vi "Filter Data.vi"(8 "error in":errorcluster, 9 "Record state change":bool=TRUE, 10 "Analyzed Data Sets":T1) -> (0 "error out":errorcluster, 1 "Send?":bool, 2 "Analyzed Data Sets Out":T1)   [LabVIEW 2018, in "File IO.lvlib"]
uses:
  File IO.lvlib
  Top Level/Shared Controls/Analyzed Data Sets.ctl
  Top Level/Shared Controls/All Data Cluster.ctl
  Top Level/Shared Controls/Acq Data.ctl
  Top Level/Shared Controls/Post-Analysis Data.ctl
  Top Level/Shared Controls/Calculated Data.ctl
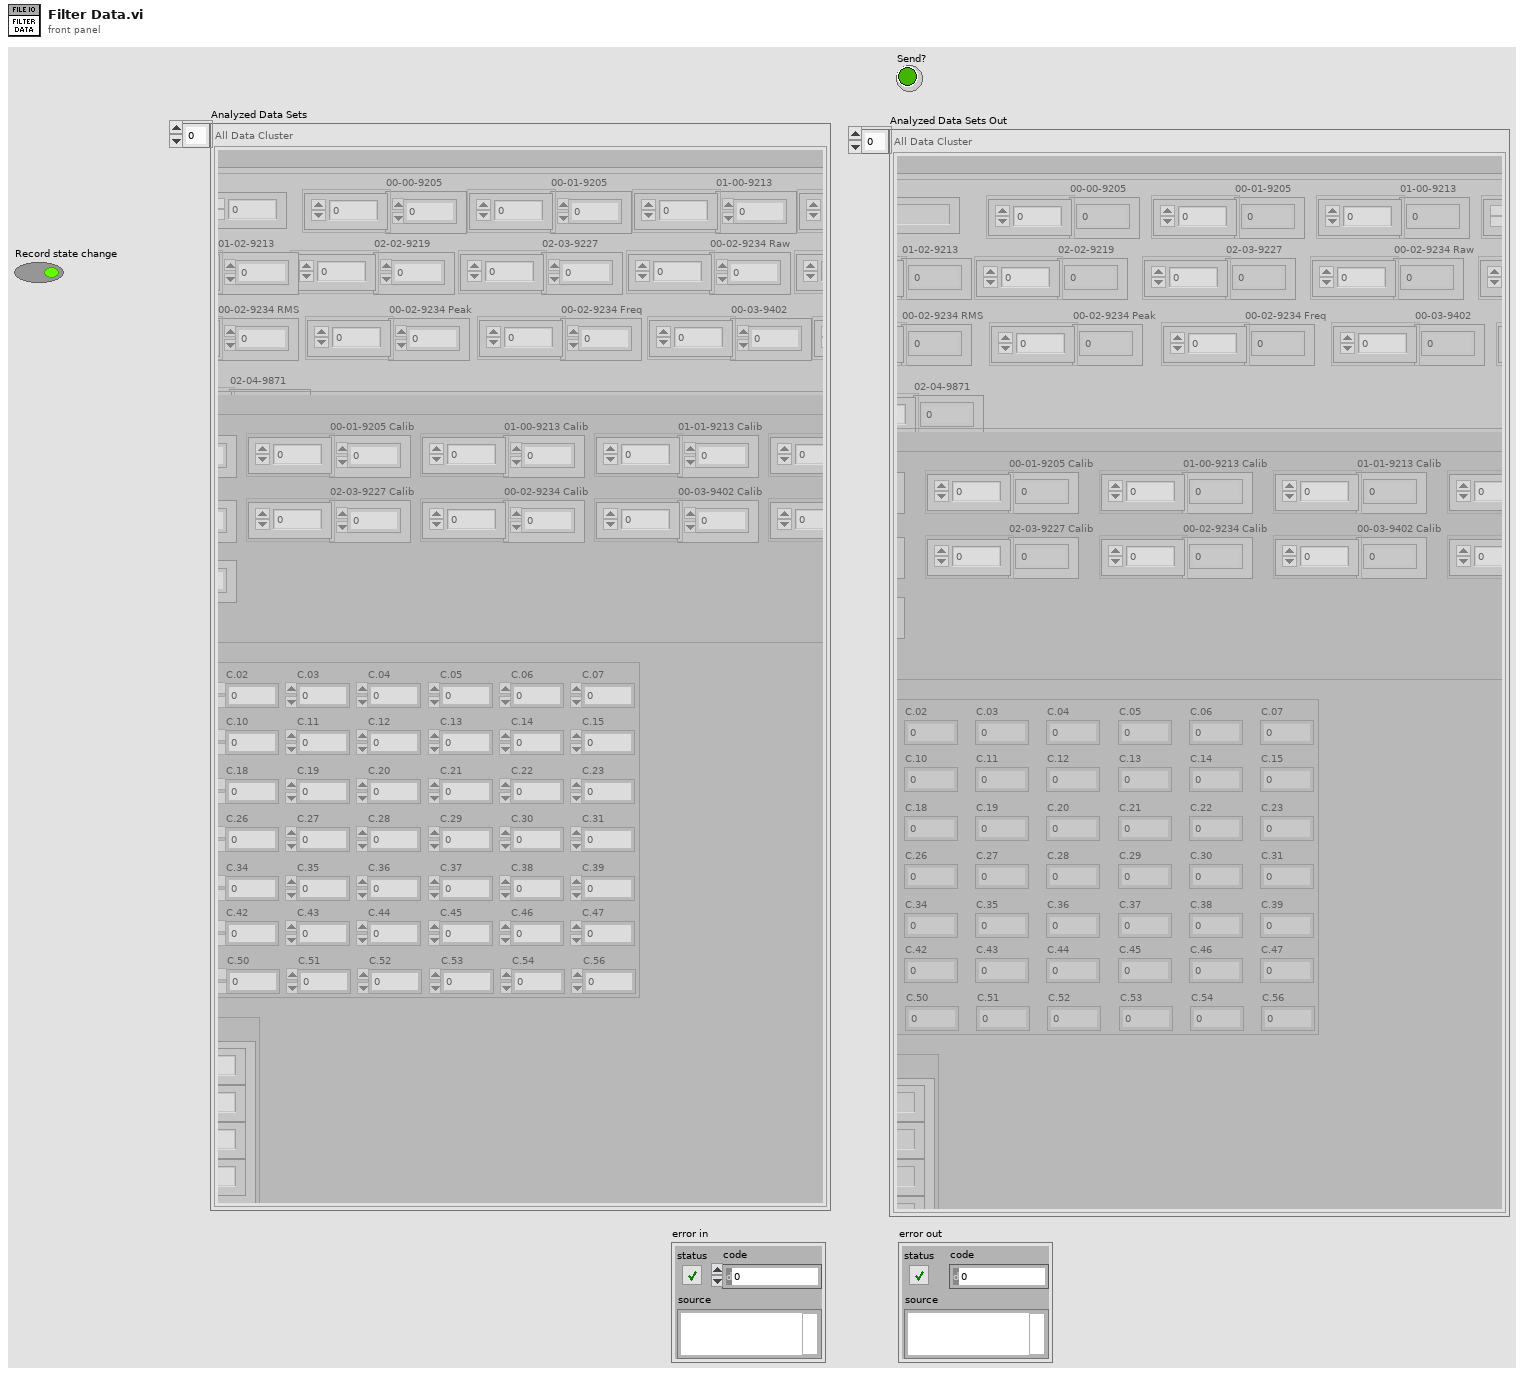
[diagram p1: front panel]
types:
  T1 = typedef "Analyzed Data Sets.ctl" = T2[]
  T2 = typedef "All Data Cluster.ctl" = cluster{"Acq Data":T3, "Post-Analysis Data":T4}
  T3 = typedef "Acq Data.ctl" = cluster{"Timestamp":timestamp, "Acq Period (ms)":i64, "00-00-9205":dbl[], "00-01-9205":dbl[], "01-00-9213":dbl[], "01-01-9213":dbl[], "01-02-9213":dbl[], "02-02-9219":dbl[], "02-03-9227":dbl[], "00-02-9234 Raw":dbl[], "00-02-9234 DC":dbl[], "00-02-9234 RMS":dbl[], "00-02-9234 Peak":dbl[], "00-02-9234 Freq":dbl[], "00-03-9402":dbl[], "02-05-9205":dbl[], "02-04-9871":dbl[]}
  T4 = typedef "Post-Analysis Data.ctl" = cluster{"Calibrated Data":cluster{"00-00-9205 Calib":dbl[], "00-01-9205 Calib":dbl[], "01-00-9213 Calib":dbl[], "01-01-9213 Calib":dbl[], "01-02-9213 Calib":dbl[], "02-02-9219 Calib":dbl[], "02-03-9227 Calib":dbl[], "00-02-9234 Calib":dbl[], "00-03-9402 Calib":dbl[], "02-05-9205 Calib":dbl[], "02-04-9871 2DArray":dbl[][]}, "Calculated Data":T5, "Indicator Data":cluster{"00-02-9234 Peak Vel (in/sec)":dbl[]}}
  T5 = typedef "Calculated Data.ctl" = cluster{"C.00":dbl, "C.01":dbl, "C.02":dbl, "C.03":dbl, "C.04":dbl, "C.05":dbl, "C.06":dbl, "C.07":dbl, "C.08":dbl, "C.09":dbl, "C.10":dbl, "C.11":dbl, "C.12":dbl, "C.13":dbl, "C.14":dbl, "C.15":dbl, "C.16":dbl, "C.17":dbl, "C.18":dbl, "C.19":dbl, "C.20":dbl, "C.21":dbl, "C.22":dbl, "C.23":dbl, "C.24":dbl, "C.25":dbl, "C.26":dbl, "C.27":dbl, "C.28":dbl, "C.29":dbl, "C.30":dbl, "C.31":dbl, "C.32":dbl, "C.33":dbl, "C.34":dbl, "C.35":dbl, "C.36":dbl, "C.37":dbl, "C.38":dbl, "C.39":dbl, "C.40":dbl, "C.41":dbl, "C.42":dbl, "C.43":dbl, "C.44":dbl, "C.45":dbl, "C.46":dbl, "C.47":dbl, "C.48":dbl, "C.49":dbl, "C.50":dbl, "C.51":dbl, "C.52":dbl, "C.53":dbl, "C.54":dbl, "C.56":dbl}
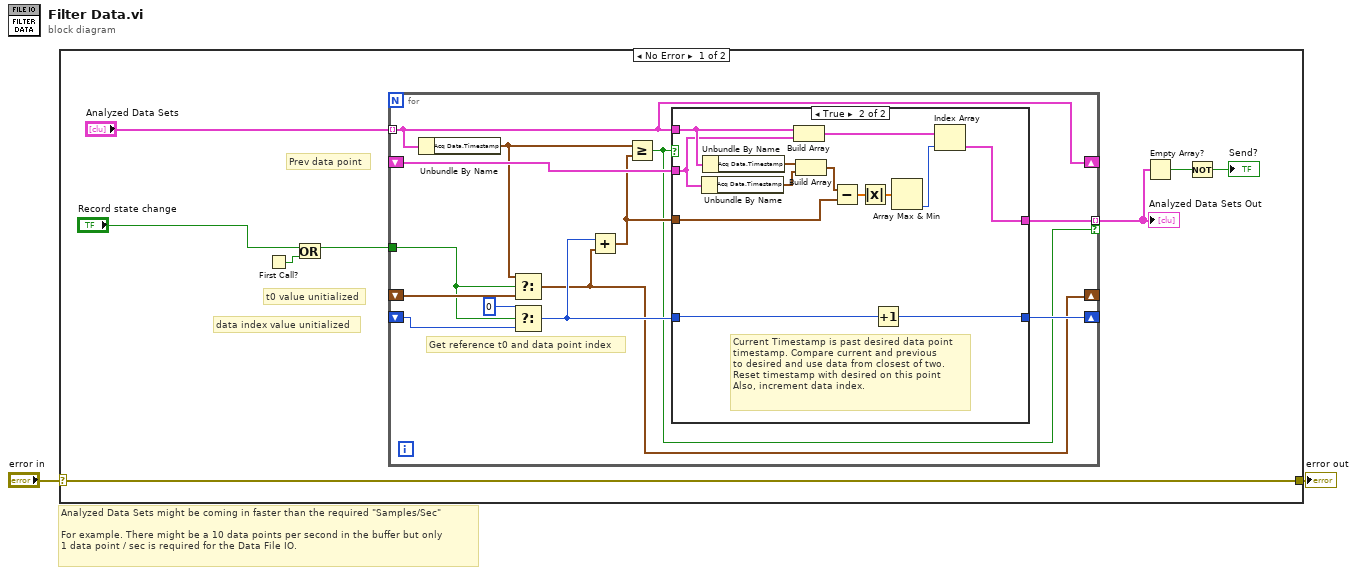
[diagram p0: block diagram]
diagram:
  # "Analyzed Data Sets might be coming in faster than the required \"Samples/Sec\"\n\nFor example. There might be a 10 data points per second in the buffer but only \n1 data point / sec is required for the Data File IO."
  n1 = case shown="No Error" "error in" {
    selector: "error in" -> [w3 w39]
    tunnel: [w3 w39] -> w1
    frame No Error {
      # "Prev data point"
      # "data index value unitialized"
      # "t0 value unitialized"
      n2 = First Call?() -> (First Call?: T/F=w5:bool)
      n3 = Or(x="Record state change", y=w5) -> (x .or. y?=w6:bool)
      n4 = for {
        tunnel: "Analyzed Data Sets" -> [w14] mode=indexing
        tunnel: w6 -> [w20]
        shift-right: [w12] -> _
        shift-left: _ -> [w23]
        shift-right: [w16] -> _
        shift-left: _ -> [w21]
        shift-right: [w14] -> _
        shift-left: _ -> [w19]
        tunnel: [w13] -> w4 mode=indexing if=w15
        # "Get reference t0 and data point index"
        n5 = Unbundle By Name(w14) -> ("Acq Data.Timestamp"=w11:timestamp)
        n6 = Select(t=w11, s=w20, f=w23) -> (s? t:f=w12:timestamp)
        n7 = Select(t=i64 0, s=w20, f=w21) -> (s? t:f=w17:i64)
        n8 = Add(x=w17, y=w12) -> (x+y=w18:timestamp)
        n9 = Greater Or Equal?(x=w11, y=w18) -> (x >= y?=w15:bool)
        n10 = case shown="True" w15 {
          tunnel: w17 -> [w25 w28]
          tunnel: w14 -> [w24 w36]
          tunnel: w19 -> [_ w35]
          tunnel: w18 -> [_ w31]
          tunnel: [w25 w27] -> w16
          tunnel: [w24 w26] -> w13
          frame False {
          }
          frame True {
            # "Current Timestamp is past desired data point\ntimestamp. Compare current and previous\nto desired and use data from closest of two.\nReset timestamp with desired on this point\nAlso, increment data index."
            n11 = Unbundle By Name(w35) -> ("Acq Data.Timestamp"=w37:timestamp)
            n12 = Unbundle By Name(w36) -> ("Acq Data.Timestamp"=w38:timestamp)
            n13 = Build Array(w36, w35) -> (w32:T2[])
            n14 = Build Array(w38, w37) -> (w30:timestamp[])
            n15 = Subtract(x=w30, y=w31) -> (x-y=w34:dbl[])
            n16 = Absolute Value(x=w34) -> (abs(x)=w33:dbl[])
            n17 = Increment(x=w28) -> (x+1=w27:i64)
            n18 = Array Max & Min(array=w33) -> (min index (indices)=w29:i32)  [unwired: 3 out]
            n19 = Index Array(array=w32, index=w29) -> (element=w26:T2)
          }
        }
      }
      "Analyzed Data Sets Out" <- w4
      n20 = Empty Array?(array=w4) -> (empty?=w9:bool)
      n21 = Not(x=w9) -> (.not. x?=→"Send?":bool)
    }
    frame Error {
    }
  }
  "error out" <- w1
